vi "Stage v2.vi"() -> ()   [LabVIEW 2025]
uses:
  upper limit.ctl
  lower limit.ctl
  libximc.lvlib
panel:
  in  "Copy Positions":bool
  out "X/256":i32
  out "Z/256":i32
  out "Y/256":i32
  in  "Zero":bool
  in  "Go Home":bool
  in  "Tab Control":T1(tab)=enum."Shift Stage"
  in  "Controller 3":u16(ring) items=["xi-com:\\\\.\\COM4", "xi-com:\\\\.\\COM5", "xi-com:\\\\.\\COM6"]
  in  "Controller 2":u16(ring) items=["xi-com:\\\\.\\COM4", "xi-com:\\\\.\\COM5", "xi-com:\\\\.\\COM6"]
  in  "Controller 1":u16(ring) items=["xi-com:\\\\.\\COM4", "xi-com:\\\\.\\COM5", "xi-com:\\\\.\\COM6"]
  out "s/n 1":u32
  out "s/n 3":u32
  out "s/n 2":u32
  in  "Destination Y":i32
  in  "Destination Z":i32
  in  "Destination X":i32
  in  "Move To Destination":bool
  in  "Update Position":bool
  in  "Move Relative":bool
  in  "Shift Y":i32
  in  "Shift Z":i32
  in  "Shift X":i32
  in  "Shift Amount (Steps)":i32
  in  "shift stage":bool
  in  "Exit":bool
  out "Cursor X":dbl format="%#.2f"
  out "Cursor Z":dbl format="%#.2f"
  out "Cursor Y":dbl format="%#.2f"
  # "Position Status"
  # "Note: units of all positions are in steps."
  # "Initializes each motor in XILab."
  # "Controller IDs"
  # "Serial Numbers"
  # "Moves individual motors to desired height (units in steps)."
  # "Moves individual motors a number of steps."
  # "Moves all three motors the same amount of steps."
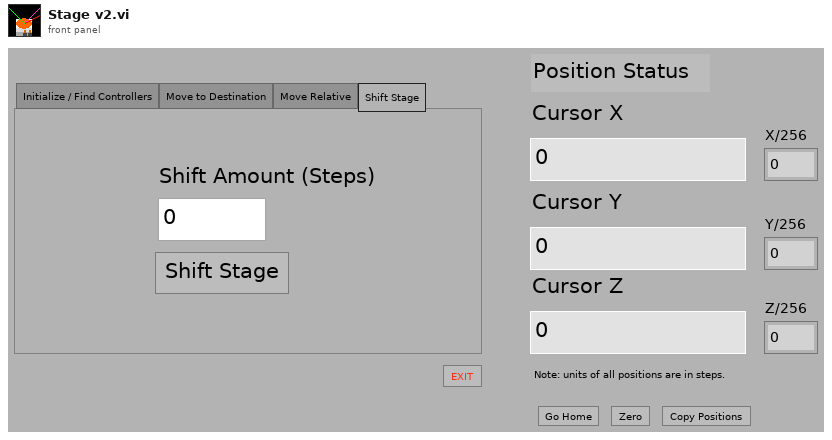
[diagram p1: front panel]
types:
  T1 = enum32{"Initialize / Find Controllers", "Move to Destination", "Move Relative", "Shift Stage"}
  T2 = enum32{"invalid app kind", "Development System", "Run Time System", "Student Edition", "Embedded LabVIEW", "Evaluation", "Custom"}
  T3 = cluster{"Number of controllers":i32, "Controllers' names":string[], "variant":variant, "quit":bool, "IDs":i32[]}
  T4 = typedef "eventvkey.ctl" = enum16{"ASCII", "Enter", "Return", "Shift", "Ctrl", "Alt", "Cmd", "Opt", "Caps", "NumLock", "Clear", "Break", "Up", "Down", "Left", "Right", "Insert", "Delete", "Home", "End", "PageUp", "PageDown", "Escape", "Help", "Pause", "ScrollLock", "F1", "F2", "F3", "F4", "F5", "F6", "F7", "F8", "F9", "F10", "F11", "F12", "F13", "F14", "F15", "F16", "F17", "F18", "F19", "F20", "F21", "F22", "F23", "F24", "Play", "VolumeUp", "VolumeDown", "Mute", "Two Byte Char"}
  T5 = typedef "lower limit.ctl" = i32
  T6 = typedef "upper limit.ctl" = i32
  T7 = cluster{"MoveSts":u32, "MvCmdSts":u32, "PWRSts":u32, "EncSts":u32, "WindSts":u32, "CurPosition":i32, "uCurPosition":i32, "@dummy control@":i8, "@dummy control@":i8, "@dummy control@":i8, "@dummy control@":i8, "EncPosition":i64, "CurSpeed":i32, "uCurSpeed":i32, "Ipwr":i32, "Upwr":i32, "Iusb":i32, "Uusb":i32, "CurT":i32, "Flags":u32, "GPIOFlags":u32, "CmdBufFreeSpace":u32}
  T8 = cluster{"Shift Y":i32, "Shift Z":i32, "Shift X":i32}
  T9 = cluster{"Destination Y":i32, "Destination Z":i32, "Destination X":i32}
  T10 = cluster{"Shift Amount (Steps)":i32, "Shift Amount (Steps)":i32, "Shift Amount (Steps)":i32}
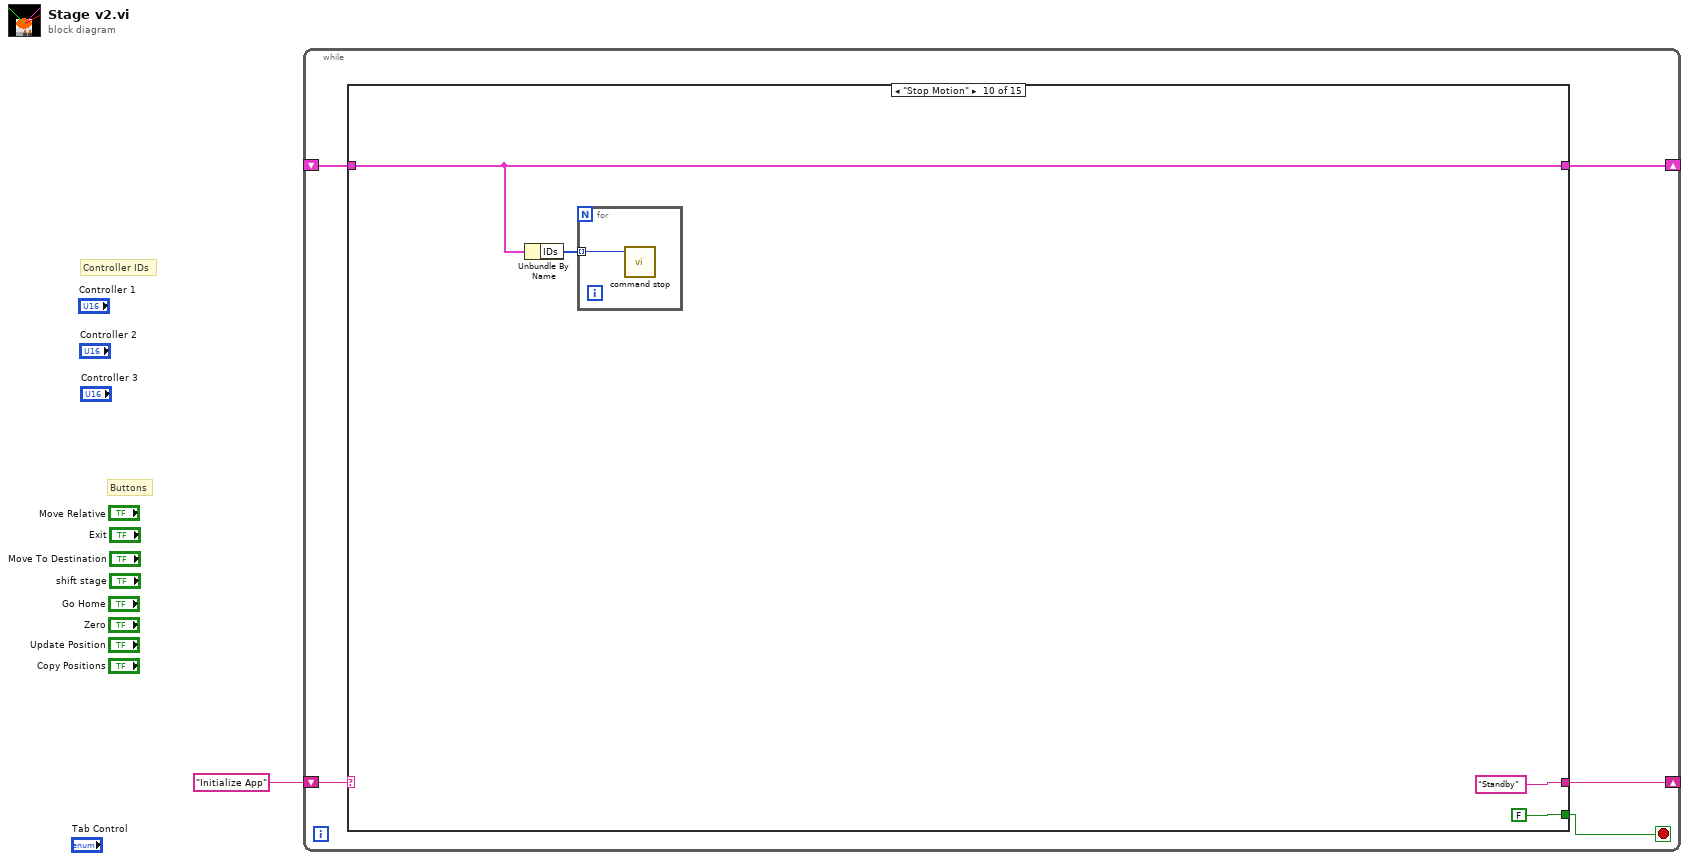
[diagram p0: block diagram]
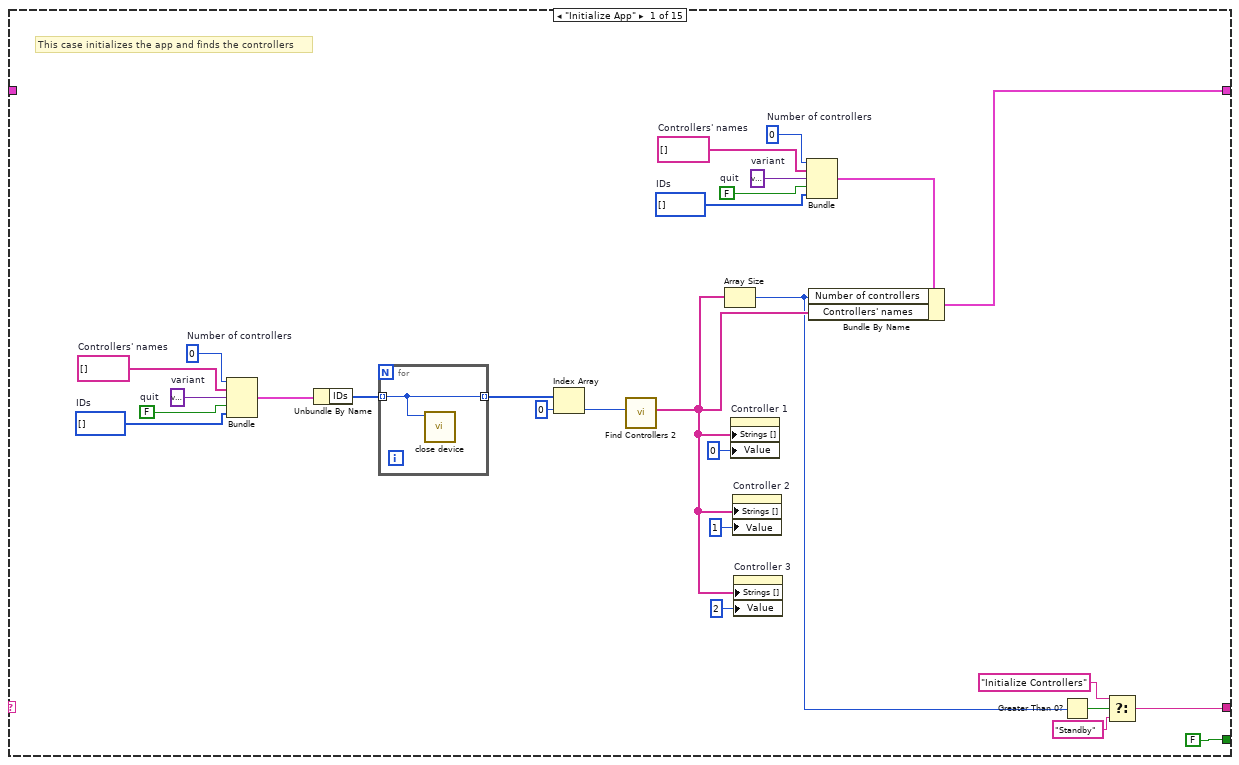
[diagram p2: hidden frame]
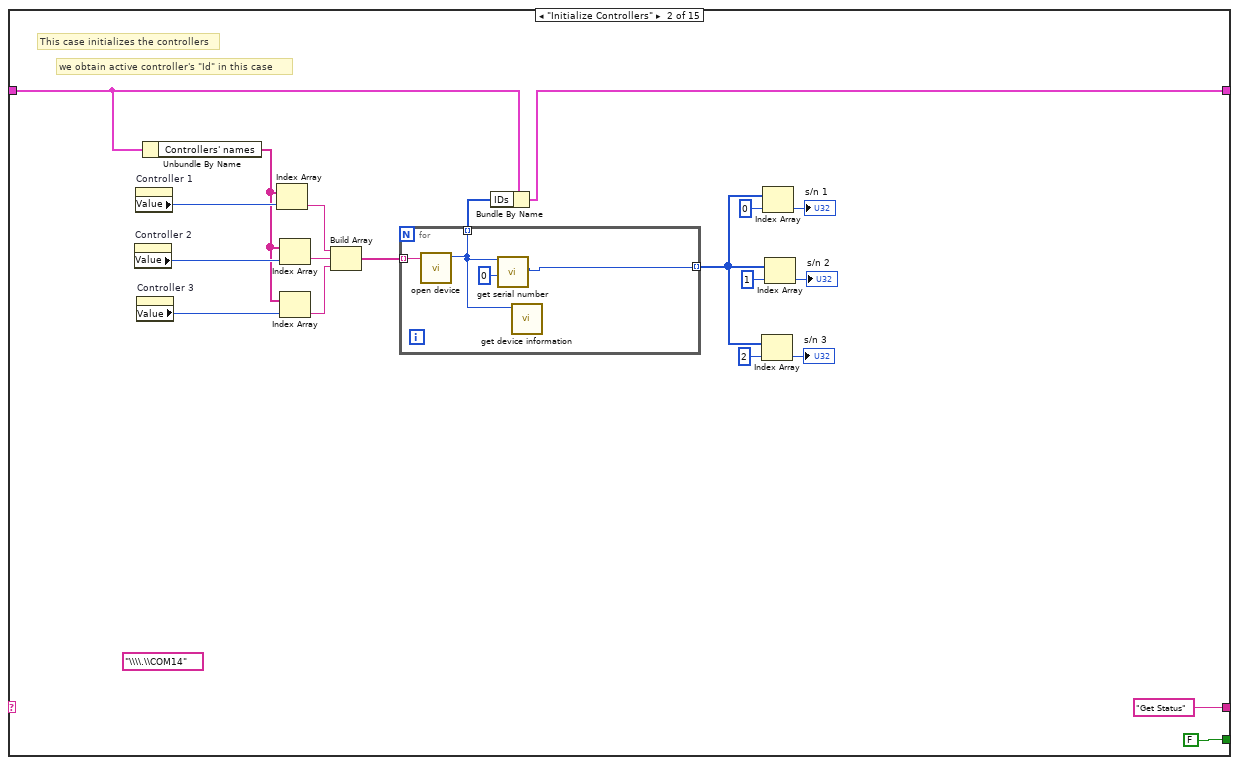
[diagram p3: hidden frame]
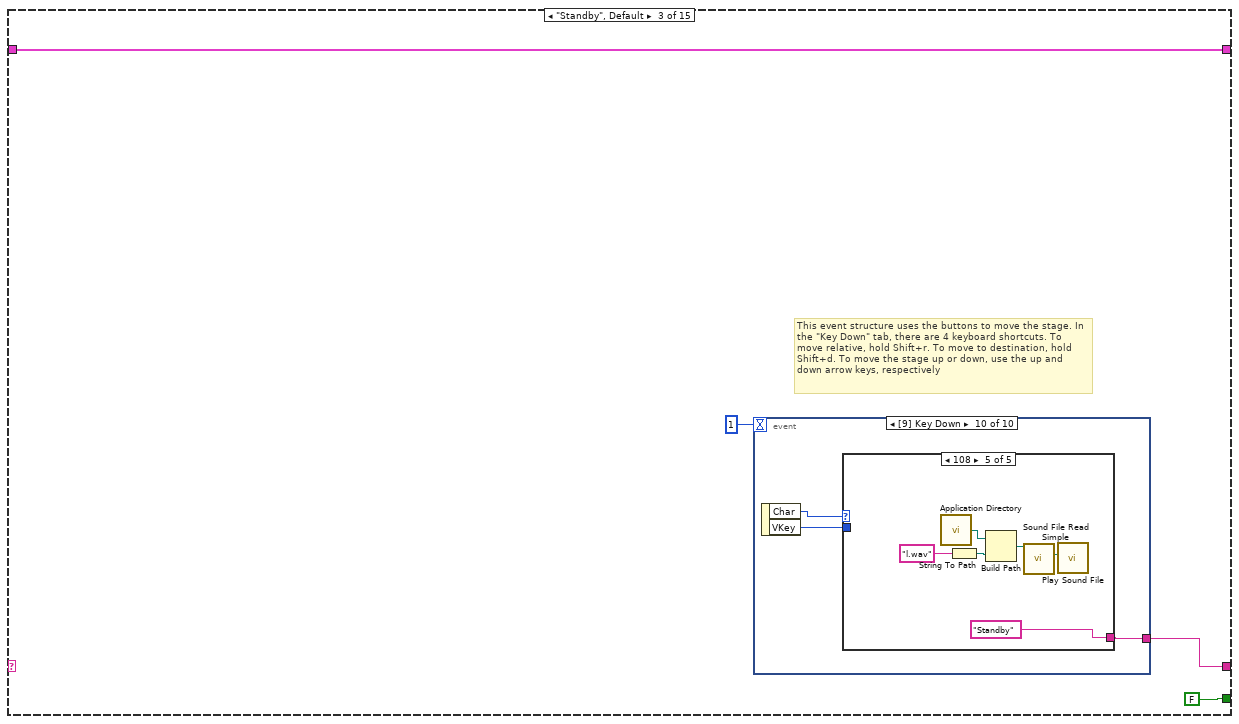
[diagram p4: hidden frame]
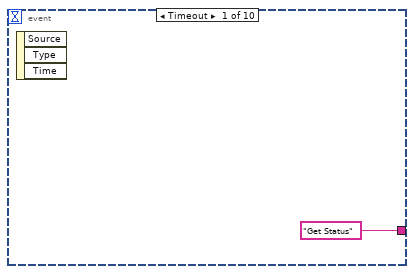
[diagram p5: hidden frame]
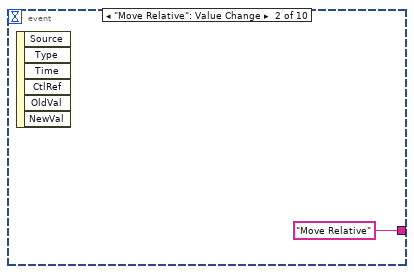
[diagram p6: hidden frame]
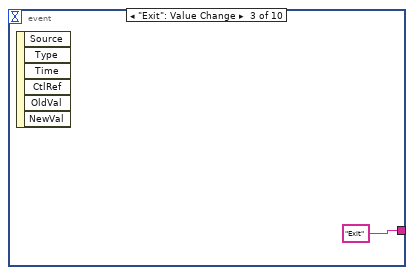
[diagram p7: hidden frame]
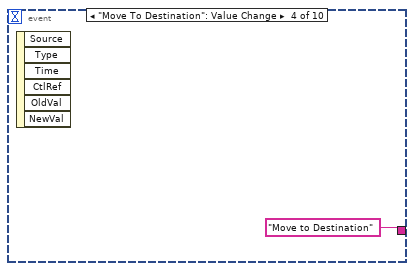
[diagram p8: hidden frame]
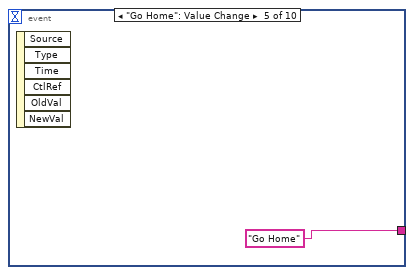
[diagram p9: hidden frame]
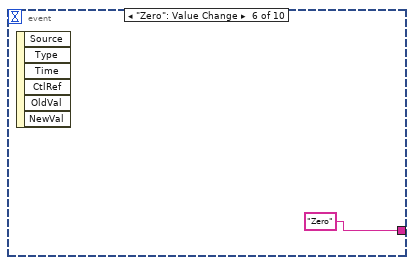
[diagram p10: hidden frame]
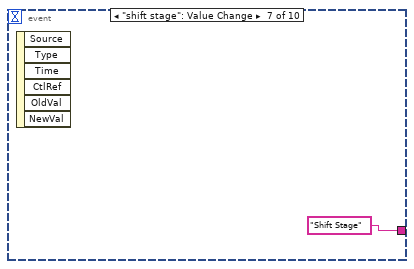
[diagram p11: hidden frame]
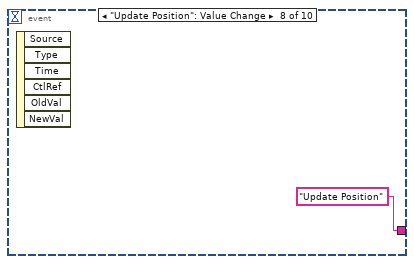
[diagram p12: hidden frame]
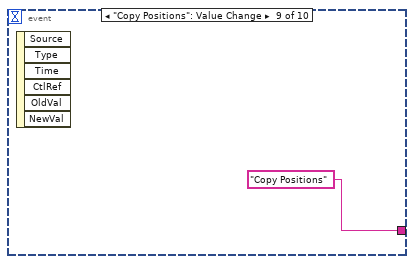
[diagram p13: hidden frame]
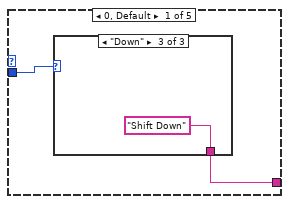
[diagram p14: hidden frame]
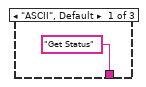
[diagram p15: hidden frame]
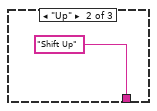
[diagram p16: hidden frame]
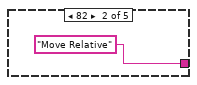
[diagram p17: hidden frame]
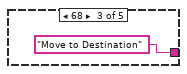
[diagram p18: hidden frame]
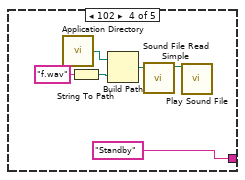
[diagram p19: hidden frame]
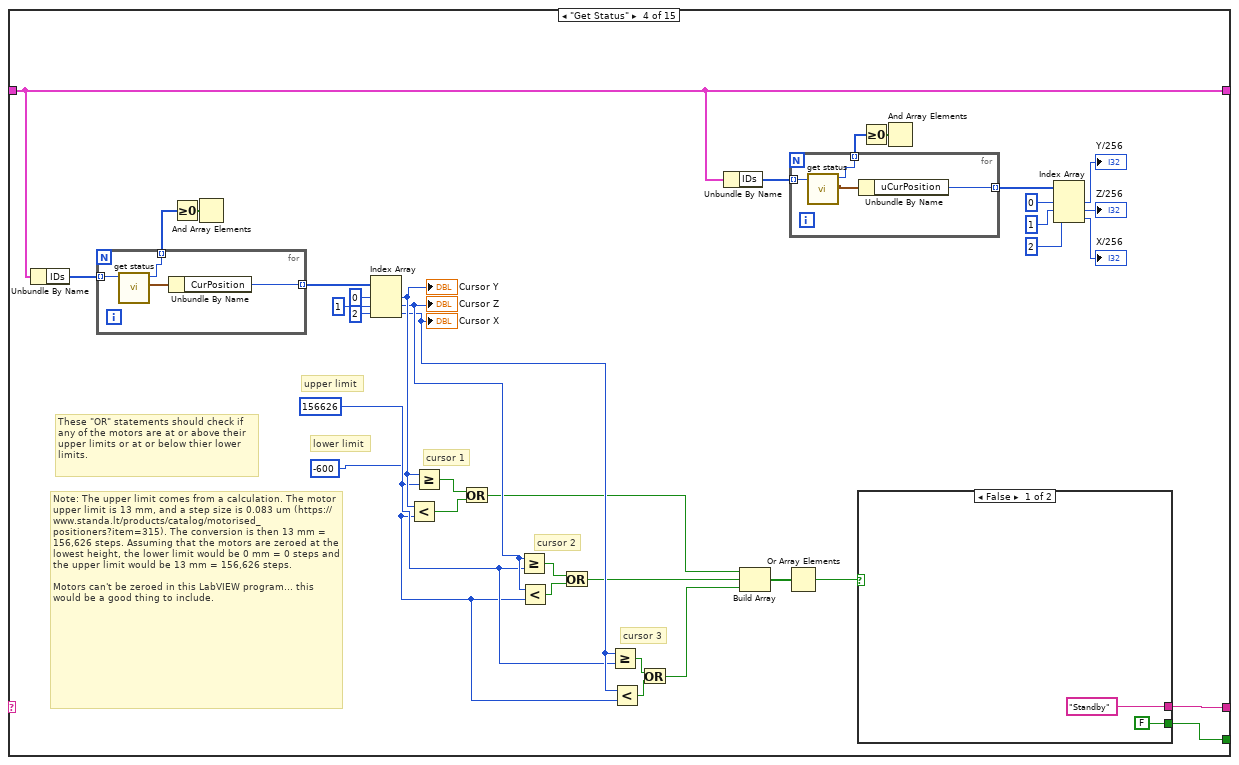
[diagram p20: hidden frame]
diagram:
  # "Buttons"
  # "Controller IDs"
  n1 = while {
    shift-right: [w5] -> _
    shift-left: _ -> [w6]
    shift-right: [w4] -> _
    shift-left: "Initialize App" -> [w3]
    stop <- w2 stop-if-true
    n2 = case shown="\"Stop Motion\"" w3 {
      tunnel: [w27 w44 w62 w94 w151 w213 w262 w320 w380 w430 w435 w440 w448 w470 w478] -> w5
      tunnel: w6 -> [_ w45 w62 w94 w151 w212 w262 w320 w380 w430 w435 w440 w448 w470 w478]
      tunnel: [w8 "Get Status" w60 w119 w150 w211 w261 w319 w379 "Standby" "Standby" "Standby" "Standby" "Standby" "Standby"] -> w4
      tunnel: [FALSE ("quit") FALSE ("quit") FALSE ("quit") w106 FALSE ("quit") FALSE ("quit") FALSE FALSE FALSE FALSE FALSE FALSE FALSE FALSE TRUE ("quit")] -> w2
      frame "Initialize App" {
        w14 = i32[] []  # IDs
        w15 = FALSE  # quit
        w16 = variant  # variant
        w17 = string[] []  # Controllers' names
        w18 = 0  # Number of controllers
        w29 = i32[] []  # IDs
        w30 = FALSE  # quit
        w31 = variant  # variant
        w32 = string[] []  # Controllers' names
        w33 = 0  # Number of controllers
        # "This case initializes the app and finds the controllers"
        n3 = Bundle("Number of controllers"=w18, "Controllers' names"=w17, "variant"=w16, "quit"=w15, "IDs"=w14) -> (w13:T3)  [unwired: 1 in]
        n4 = Unbundle By Name(w13) -> ("IDs"=w20:i32[])
        n5 = for {
          tunnel: w20 -> [w34] mode=indexing
          tunnel: [w34] -> w19 mode=indexing
          n6 = call "close device.vi"("id"=w34) -> ()  [unwired: 8 in, 3 out]
        }
        n7 = Index Array(array=w19, index=0) -> (element=w25:i32)
        n8 = call "Find Controllers 2.vi"("Numeric"=w25) -> ("Names"=w21:string[])  [unwired: 9 in, 1 out]
        n9 = Array Size(array=w21) -> (size(s)=w11:i32)
        n10 = property on="Controller 1" class="Ring (strict)"("Strings []"=w21, "Value"=0) -> ()  [unwired: 2 in, 2 out]
        n11 = property on="Controller 2" class="Ring (strict)"("Strings []"=w21, "Value"=1) -> ()  [unwired: 2 in, 2 out]
        n12 = property on="Controller 3" class="Ring (strict)"("Strings []"=w21, "Value"=2 ("Controller 3")) -> ()  [unwired: 2 in, 2 out]
        n13 = Bundle("Number of controllers"=w33, "Controllers' names"=w32, "variant"=w31, "quit"=w30, "IDs"=w29) -> (w28:T3)  [unwired: 1 in]
        n14 = Bundle By Name(cluster=w28, "Number of controllers"=w11, "Controllers' names"=w21) -> (w27:T3)
        n15 = Greater Than 0?(x=w11) -> (x > 0?=w12:bool)
        n16 = Select(t="Initialize Controllers", s=w12, f="Standby") -> (s? t:f=w8:string)
      }
      frame "Initialize Controllers" {
        (unwired) "\\\\.\\COM14" ("name")
        # "we obtain active controller's \"Id\" in this case"
        # "This case initializes the controllers"
        n17 = property on="Controller 2" class="Ring (strict)"() -> ("Value"=w53:u16)  [unwired: 2 in, 2 out]
        n18 = property on="Controller 1" class="Ring (strict)"() -> ("Value"=w54:u16)  [unwired: 2 in, 2 out]
        n19 = property on="Controller 3" class="Ring (strict)"() -> ("Value"=w52:u16)  [unwired: 2 in, 2 out]
        n20 = Unbundle By Name(w45) -> ("Controllers' names"=w48:string[])
        n21 = Index Array(array=w48, index=w54) -> (element=w49:string)
        n22 = Index Array(array=w48, index=w53) -> (element=w50:string)
        n23 = Index Array(array=w48, index=w52) -> (element=w51:string)
        n24 = Build Array(w49, w50, w51) -> (w47:string[])
        n25 = for {
          tunnel: w47 -> [w58] mode=indexing
          tunnel: [w56] -> w46 mode=indexing
          tunnel: [w55] -> w37 mode=indexing
          n26 = call "open device.vi"("uri"=w58) -> ("function return"=w56:i32)  [unwired: 9 in, 1 out]
          n27 = call "get serial number.vi"("SerialNumber"=0, "id"=w56) -> ("SerialNumber out"=w55:u32)  [unwired: 7 in, 2 out]
          n28 = call "get device information.vi"("id"=w56) -> ()  [unwired: 8 in, 3 out]
        }
        n29 = Bundle By Name(cluster=w45, "IDs"=w46) -> (w44:T3)
        n30 = Index Array(array=w37, index=u32 2 ("serial")) -> (element=→"s/n 3":u32)
        n31 = Index Array(array=w37, index=u32 0 ("serial")) -> (element=→"s/n 1":u32)
        n32 = Index Array(array=w37, index=u32 1 ("serial")) -> (element=→"s/n 2":u32)
      }
      frame "Standby", Default {
        # "This event structure uses the buttons to move the stage. In the \"Key Down\" tab, there are 4 keyboard shortcuts. To move relative, hold Shift+r. To move to destination, hold Shift+d. To move the stage up or down, use the up and down arrow keys, respectively"
        n33 = event shown="[9] Key Down" {
          selector: _ -> [_ _ _ _ _ _ _ _ _ _]
          dyn-events: _ -> [_ _ _ _ _ _ _ _ _ _]
          timeout: 1 -> [_ _ _ _ _ _ _ _ _ _]
          tunnel: ["Get Status" "Move Relative" "Exit" "Move to Destination" "Go Home" "Zero" "Shift Stage" "Update Position" "Copy Positions" w74] -> w60
          event Timeout {
            n34 = event-data() -> ()  [unwired: 1 in, 3 out]
          }
          event "Move Relative": Value Change {
            n35 = event-data() -> ()  [unwired: 1 in, 6 out]
          }
          event "Exit": Value Change {
            n36 = event-data() -> ()  [unwired: 1 in, 6 out]
          }
          event "Move To Destination": Value Change {
            n37 = event-data() -> ()  [unwired: 1 in, 6 out]
          }
          event "Go Home": Value Change {
            n38 = event-data() -> ()  [unwired: 1 in, 6 out]
          }
          event "Zero": Value Change {
            n39 = event-data() -> ()  [unwired: 1 in, 6 out]
          }
          event "shift stage": Value Change {
            n40 = event-data() -> ()  [unwired: 1 in, 6 out]
          }
          event "Update Position": Value Change {
            n41 = event-data() -> ()  [unwired: 1 in, 6 out]
          }
          event "Copy Positions": Value Change {
            n42 = event-data() -> ()  [unwired: 1 in, 6 out]
          }
          event Key Down {
            n43 = event-data() -> ("Char"=w73:i16, "VKey"=w72:T4)  [unwired: 1 in]
            n44 = case shown="108" w73 {
              tunnel: [w75 "Move Relative" "Move to Destination" "Standby" "Standby"] -> w74
              tunnel: w72 -> [w76 _ _ _ _]
              frame 0, Default {
                n45 = case shown="\"Down\"" w76 {
                  tunnel: ["Get Status" "Shift Up" "Shift Down"] -> w75
                  frame "ASCII", Default {
                  }
                  frame "Up" {
                  }
                  frame "Down" {
                  }
                }
              }
              frame 82 {
              }
              frame 68 {
              }
              frame 102 {
                n46 = call <vilib>:"Application Directory.vi"() -> ("Application Directory"=w86:path)
                n47 = String To Path(string="f.wav") -> (path=w84:path)
                n48 = Build Path(base path=w86, name or relative path=w84) -> (appended path=w83:path)
                n49 = call <vilib>:"Sound File Read Simple.vi"("path"=w83) -> ("path out"=w82:path)  [unwired: 7 in, 3 out]
                n50 = call <vilib>:"Play Sound File.vi"("path"=w82) -> ()  [unwired: 9 in, 2 out]
              }
              frame 108 {
                n51 = call <vilib>:"Application Directory.vi"() -> ("Application Directory"=w92:path)
                n52 = String To Path(string="l.wav") -> (path=w90:path)
                n53 = Build Path(base path=w92, name or relative path=w90) -> (appended path=w89:path)
                n54 = call <vilib>:"Sound File Read Simple.vi"("path"=w89) -> ("path out"=w88:path)  [unwired: 7 in, 3 out]
                n55 = call <vilib>:"Play Sound File.vi"("path"=w88) -> ()  [unwired: 9 in, 2 out]
              }
            }
          }
        }
      }
      frame "Get Status" {
        w105 = T5 -600
        w107 = T6 156626
        # "cursor 3"
        # "cursor 2"
        # "cursor 1"
        # "lower limit"
        # "upper limit"
        # "Note: The upper limit comes from a calculation. The motor upper limit is 13 mm, and a step size is 0.083 um (https://www.standa.lt/products/catalog/motorised_positioners?item=315). The conversion is then 13 mm = 156,626 steps. Assuming that the motors are zeroed at the lowest height, the lower limit would be 0 mm = 0 steps and the upper limit would be 13 mm = 156,626 steps.\n\nMotors can't be zeroed in this LabVIEW program... this would be a good thing to include."
        # "These \"OR\" statements should check if any of the motors are at or above their upper limits or at or below thier lower limits."
        n56 = Unbundle By Name(w94) -> ("IDs"=w129:i32[])
        n57 = for {
          tunnel: [w147] -> w127 mode=indexing
          tunnel: w129 -> [w146] mode=indexing
          tunnel: [w145] -> w128 mode=indexing
          n58 = call "get status.vi"("id"=w146) -> ("status out"=w144:T7, "function return"=w145:i32)  [unwired: 8 in, 1 out]
          n59 = Unbundle By Name(w144) -> ("CurPosition"=w147:i32)
        }
        n60 = Greater Or Equal To 0?(x=w128) -> (x >= 0?=w123:bool[])
        n61 = And Array Elements(Boolean array=w123) -> ()  [unwired: 1 out]
        n62 = Index Array(array=w127, index #1=0 ("index"), index #2=1 ("index"), index #3=2 ("index")) -> (element #1=w121:i32, element #2=w114:i32, element #3=w113:i32)
        "Cursor Y" <- w121
        "Cursor Z" <- w114
        "Cursor X" <- w113
        n63 = Less?(x=w121, y=w105) -> (x < y?=w120:bool)
        n64 = Greater Or Equal?(x=w121, y=w107) -> (x >= y?=w122:bool)
        n65 = Or(x=w122, y=w120) -> (x .or. y?=w112:bool)
        n66 = Greater Or Equal?(x=w114, y=w107) -> (x >= y?=w118:bool)
        n67 = Less?(x=w114, y=w105) -> (x < y?=w117:bool)
        n68 = Or(x=w118, y=w117) -> (x .or. y?=w111:bool)
        n69 = Greater Or Equal?(x=w113, y=w107) -> (x >= y?=w116:bool)
        n70 = Less?(x=w113, y=w105) -> (x < y?=w115:bool)
        n71 = Or(x=w116, y=w115) -> (x .or. y?=w110:bool)
        n72 = Unbundle By Name(w94) -> ("IDs"=w104:i32[])
        n73 = Build Array(w112, w111, w110) -> (w109:bool[])
        n74 = Or Array Elements(Boolean array=w109) -> (logical OR=w108:bool)
        n75 = for {
          tunnel: [w133] -> w102 mode=indexing
          tunnel: w104 -> [w132] mode=indexing
          tunnel: [w131] -> w103 mode=indexing
          n76 = call "get status.vi"("id"=w132) -> ("status out"=w130:T7, "function return"=w131:i32)  [unwired: 8 in, 1 out]
          n77 = Unbundle By Name(w130) -> ("uCurPosition"=w133:i32)
        }
        n78 = case shown="False" w108 {
          tunnel: ["Standby" "Stop Motion"] -> w119
          tunnel: [FALSE w141] -> w106
          frame False {
          }
          frame True {
            # "If any of them move past the limits, the program will stop. You won't be able to use this LabVIEW program until the height is fixed in XILab."
            n79 = call <vilib>:"Application Directory.vi"() -> ("Application Directory"=w140:path)
            n80 = String To Path(string="l.wav") -> (path=w138:path)
            n81 = Build Path(base path=w140, name or relative path=w138) -> (appended path=w137:path)
            n82 = call <vilib>:"Sound File Read Simple.vi"("path"=w137) -> ("path out"=w136:path)  [unwired: 7 in, 3 out]
            n83 = call <vilib>:"Play Sound File.vi"("path"=w136) -> ()  [unwired: 9 in, 2 out]
            n84 = One Button Dialog(message="You've gone too far this time...\nPlease check the height of the stage and move it back to a normal height using XILab <3") -> (true=w141:bool)  [unwired: 1 in]
          }
        }
        n85 = Greater Or Equal To 0?(x=w103) -> (x >= 0?=w101:bool[])
        n86 = And Array Elements(Boolean array=w101) -> ()  [unwired: 1 out]
        n87 = Index Array(array=w102, index #1=0 ("index"), index #2=1 ("index"), index #3=2 ("index")) -> (element #1=→"Y/256":i32, element #2=→"Z/256":i32, element #3=→"X/256":i32)
      }
      frame "Move Relative" {
        w148 = T6 156626
        w149 = -1
        # "cursor 3"
        # "cursor 2"
        # "cursor 1"
        # "lower limit"
        # "upper limit"
        n88 = Unbundle By Name(w151) -> ("IDs"=w178:i32[])
        n89 = for {
          tunnel: [w205] -> w176 mode=indexing
          tunnel: w178 -> [w204] mode=indexing
          tunnel: [w203] -> w177 mode=indexing
          n90 = call "get status.vi"("id"=w204) -> ("status out"=w202:T7, "function return"=w203:i32)  [unwired: 8 in, 1 out]
          n91 = Unbundle By Name(w202) -> ("CurPosition"=w205:i32)
        }
        n92 = Greater Or Equal To 0?(x=w177) -> (x >= 0?=w172:bool[])
        n93 = And Array Elements(Boolean array=w172) -> ()  [unwired: 1 out]
        n94 = Index Array(array=w176, index #1=0 ("index"), index #2=1 ("index"), index #3=2 ("index")) -> (element #1=w160:i32, element #2=w159:i32, element #3=w158:i32)
        n95 = Add(x="Shift Y", y=w160) -> (x+y=w157:i32)
        n96 = Add(x="Shift Z", y=w159) -> (x+y=w155:i32)
        n97 = Add(x="Shift X", y=w158) -> (x+y=w156:i32)
        n98 = Less Or Equal?(x=w157, y=w149) -> (x <= y?=w170:bool)
        n99 = Greater Or Equal?(x=w156, y=w148) -> (x >= y?=w167:bool)
        n100 = Greater Or Equal?(x=w157, y=w148) -> (x >= y?=w171:bool)
        n101 = Greater Or Equal?(x=w155, y=w148) -> (x >= y?=w169:bool)
        n102 = Less Or Equal?(x=w155, y=w149) -> (x <= y?=w168:bool)
        n103 = Less Or Equal?(x=w156, y=w149) -> (x <= y?=w166:bool)
        n104 = Or(x=w167, y=w166) -> (x .or. y?=w163:bool)
        n105 = Or(x=w169, y=w168) -> (x .or. y?=w164:bool)
        n106 = Or(x=w171, y=w170) -> (x .or. y?=w165:bool)
        n107 = Build Array(w165, w164, w163) -> (w162:bool[])
        n108 = Or Array Elements(Boolean array=w162) -> (logical OR=w161:bool)
        n109 = case shown="False" w161 {
          tunnel: ["Standby" "Stop Motion"] -> w150
          tunnel: "Shift Y" -> [w190 _]
          tunnel: "Shift Z" -> [w189 _]
          tunnel: "Shift X" -> [w188 _]
          tunnel: w151 -> [w187 w199]
          tunnel: [w185 w199] -> _
          frame False {
            n110 = Bundle("Shift Y"=w190, "Shift Z"=w189, "Shift X"=w188) -> (w186:T8)  [unwired: 1 in]
            n111 = Bundle By Name(cluster=w187, "variant"=w186) -> (w185:T3)
            n112 = Unbundle By Name(w185) -> ("IDs"=w180:i32[], "variant"=w182:variant)
            n113 = Variant To Data(type=cluster{u32, u32, u32} {0, 0, 0}, Variant=w182) -> (data=w183:cluster{u32, u32, u32})  [unwired: 1 in, 1 out]
            n114 = Cluster To Array(cluster=w183) -> (array=w184:u32[])
            n115 = for {
              tunnel: w184 -> [w192] mode=indexing
              tunnel: w180 -> [w193] mode=indexing
              n116 = call "command movr.vi"("DeltaPosition"=w192, "id"=w193) -> ()  [unwired: 8 in, 2 out]
            }
          }
          frame True {
            # "If any of them move past the limits, the motors won't move."
            n117 = call <vilib>:"Application Directory.vi"() -> ("Application Directory"=w198:path)
            n118 = String To Path(string="l.wav") -> (path=w196:path)
            n119 = Build Path(base path=w198, name or relative path=w196) -> (appended path=w195:path)
            n120 = call <vilib>:"Sound File Read Simple.vi"("path"=w195) -> ("path out"=w194:path)  [unwired: 7 in, 3 out]
            n121 = One Button Dialog(message="You've gone too far this time...\nPlease ensure the step size does not go past the limits <3") -> ()  [unwired: 1 in, 1 out]
            n122 = call <vilib>:"Play Sound File.vi"("path"=w194) -> ()  [unwired: 9 in, 2 out]
          }
        }
      }
      frame "Move to Destination" {
        w206 = T6 156626
        w207 = -1
        # "cursor 3"
        # "cursor 2"
        # "cursor 1"
        # "lower limit"
        # "upper limit"
        n123 = Unbundle By Name(w212) -> ("IDs"=w231:i32[])
        n124 = for {
          tunnel: [w258] -> w229 mode=indexing
          tunnel: w231 -> [w257] mode=indexing
          tunnel: [w256] -> w230 mode=indexing
          n125 = call "get status.vi"("id"=w257) -> ("status out"=w255:T7, "function return"=w256:i32)  [unwired: 8 in, 1 out]
          n126 = Unbundle By Name(w255) -> ("CurPosition"=w258:i32)
        }
        n127 = Greater Or Equal To 0?(x=w230) -> (x >= 0?=w225:bool[])
        n128 = And Array Elements(Boolean array=w225) -> ()  [unwired: 1 out]
        n129 = Index Array(array=w229, index #1=0 ("index"), index #2=1 ("index"), index #3=2 ("index")) -> ()  [unwired: 3 out]
        n130 = Less Or Equal?(x="Destination Y", y=w207) -> (x <= y?=w223:bool)
        n131 = Greater Or Equal?(x="Destination X", y=w206) -> (x >= y?=w220:bool)
        n132 = Greater Or Equal?(x="Destination Y", y=w206) -> (x >= y?=w224:bool)
        n133 = Greater Or Equal?(x="Destination Z", y=w206) -> (x >= y?=w222:bool)
        n134 = Less Or Equal?(x="Destination Z", y=w207) -> (x <= y?=w221:bool)
        n135 = Less Or Equal?(x="Destination X", y=w207) -> (x <= y?=w219:bool)
        n136 = Or(x=w220, y=w219) -> (x .or. y?=w216:bool)
        n137 = Or(x=w222, y=w221) -> (x .or. y?=w217:bool)
        n138 = Or(x=w224, y=w223) -> (x .or. y?=w218:bool)
        n139 = Build Array(w218, w217, w216) -> (w215:bool[])
        n140 = Or Array Elements(Boolean array=w215) -> (logical OR=w214:bool)
        n141 = case shown="False" w214 {
          tunnel: ["Standby" "Stop Motion"] -> w211
          tunnel: "Destination Y" -> [w237 _]
          tunnel: "Destination Z" -> [w236 _]
          tunnel: "Destination X" -> [w235 _]
          tunnel: w212 -> [w234 w252]
          tunnel: [w233 w252] -> w213
          frame False {
            n142 = Bundle("Destination Y"=w237, "Destination Z"=w236, "Destination X"=w235) -> (w239:T9)  [unwired: 1 in]
            n143 = Bundle By Name(cluster=w234, "variant"=w239) -> (w233:T3)
            n144 = Unbundle By Name(w233) -> ("IDs"=w241:i32[], "variant"=w243:variant)
            n145 = Variant To Data(type=cluster{u32, u32, u32} {0, 0, 0}, Variant=w243) -> (data=w240:cluster{u32, u32, u32})  [unwired: 1 in, 1 out]
            n146 = Cluster To Array(cluster=w240) -> (array=w242:u32[])
            n147 = for {
              tunnel: w242 -> [w245] mode=indexing
              tunnel: w241 -> [w246] mode=indexing
              n148 = call "command move.vi"("Position"=w245, "id"=w246) -> ()  [unwired: 8 in, 2 out]
            }
          }
          frame True {
            # "If any of them move past the limits, the motors won't move."
            n149 = call <vilib>:"Application Directory.vi"() -> ("Application Directory"=w251:path)
            n150 = String To Path(string="l.wav") -> (path=w249:path)
            n151 = Build Path(base path=w251, name or relative path=w249) -> (appended path=w248:path)
            n152 = call <vilib>:"Sound File Read Simple.vi"("path"=w248) -> ("path out"=w247:path)  [unwired: 7 in, 3 out]
            n153 = call <vilib>:"Play Sound File.vi"("path"=w247) -> ()  [unwired: 9 in, 2 out]
            n154 = One Button Dialog(message="You've gone too far this time...\nPlease ensure the step size does not go past the limits <3") -> ()  [unwired: 1 in, 1 out]
          }
        }
      }
      frame "Shift Stage" {
        w259 = T6 156626
        w260 = -1
        # "cursor 3"
        # "cursor 2"
        # "cursor 1"
        # "lower limit"
        # "upper limit"
        n155 = Unbundle By Name(w262) -> ("IDs"=w287:i32[])
        n156 = for {
          tunnel: [w314] -> w285 mode=indexing
          tunnel: w287 -> [w313] mode=indexing
          tunnel: [w312] -> w286 mode=indexing
          n157 = call "get status.vi"("id"=w313) -> ("status out"=w311:T7, "function return"=w312:i32)  [unwired: 8 in, 1 out]
          n158 = Unbundle By Name(w311) -> ("CurPosition"=w314:i32)
        }
        n159 = Greater Or Equal To 0?(x=w286) -> (x >= 0?=w281:bool[])
        n160 = And Array Elements(Boolean array=w281) -> ()  [unwired: 1 out]
        n161 = Index Array(array=w285, index #1=0 ("index"), index #2=1 ("index"), index #3=2 ("index")) -> (element #1=w269:i32, element #2=w268:i32, element #3=w267:i32)
        n162 = Add(x="Shift Amount (Steps)", y=w269) -> (x+y=w266:i32)
        n163 = Add(x="Shift Amount (Steps)", y=w268) -> (x+y=w264:i32)
        n164 = Add(x="Shift Amount (Steps)", y=w267) -> (x+y=w265:i32)
        n165 = Less Or Equal?(x=w266, y=w260) -> (x <= y?=w279:bool)
        n166 = Greater Or Equal?(x=w265, y=w259) -> (x >= y?=w276:bool)
        n167 = Greater Or Equal?(x=w266, y=w259) -> (x >= y?=w280:bool)
        n168 = Greater Or Equal?(x=w264, y=w259) -> (x >= y?=w278:bool)
        n169 = Less Or Equal?(x=w264, y=w260) -> (x <= y?=w277:bool)
        n170 = Less Or Equal?(x=w265, y=w260) -> (x <= y?=w275:bool)
        n171 = Or(x=w276, y=w275) -> (x .or. y?=w272:bool)
        n172 = Or(x=w278, y=w277) -> (x .or. y?=w273:bool)
        n173 = Or(x=w280, y=w279) -> (x .or. y?=w274:bool)
        n174 = Build Array(w274, w273, w272) -> (w271:bool[])
        n175 = Or Array Elements(Boolean array=w271) -> (logical OR=w270:bool)
        n176 = case shown="False" w270 {
          tunnel: ["Standby" "Stop Motion"] -> w261
          tunnel: "Shift Amount (Steps)" -> [w299 _]
          tunnel: "Shift Amount (Steps)" -> [w298 _]
          tunnel: "Shift Amount (Steps)" -> [w297 _]
          tunnel: w262 -> [w296 w308]
          tunnel: [w294 w308] -> _
          frame False {
            n177 = Bundle("Shift Amount (Steps)"=w299, "Shift Amount (Steps)"=w298, "Shift Amount (Steps)"=w297) -> (w295:T10)  [unwired: 1 in]
            n178 = Bundle By Name(cluster=w296, "variant"=w295) -> (w294:T3)
            n179 = Unbundle By Name(w294) -> ("IDs"=w289:i32[], "variant"=w291:variant)
            n180 = Variant To Data(type=cluster{u32, u32, u32} {0, 0, 0}, Variant=w291) -> (data=w292:cluster{u32, u32, u32})  [unwired: 1 in, 1 out]
            n181 = Cluster To Array(cluster=w292) -> (array=w293:u32[])
            n182 = for {
              tunnel: w293 -> [w301] mode=indexing
              tunnel: w289 -> [w302] mode=indexing
              n183 = call "command movr.vi"("DeltaPosition"=w301, "id"=w302) -> ()  [unwired: 8 in, 2 out]
            }
          }
          frame True {
            # "If any of them move past the limits, the motors won't move."
            n184 = call <vilib>:"Application Directory.vi"() -> ("Application Directory"=w307:path)
            n185 = String To Path(string="l.wav") -> (path=w305:path)
            n186 = Build Path(base path=w307, name or relative path=w305) -> (appended path=w304:path)
            n187 = call <vilib>:"Sound File Read Simple.vi"("path"=w304) -> ("path out"=w303:path)  [unwired: 7 in, 3 out]
            n188 = call <vilib>:"Play Sound File.vi"("path"=w303) -> ()  [unwired: 9 in, 2 out]
            n189 = One Button Dialog(message="You've gone too far this time...\nPlease ensure the step size does not go past the limits <3") -> ()  [unwired: 1 in, 1 out]
          }
        }
      }
      frame "Shift Up" {
        w315 = T6 156626
        w316 = -1
        # "cursor 3"
        # "cursor 2"
        # "cursor 1"
        # "lower limit"
        # "upper limit"
        n190 = Unbundle By Name(w320) -> ("IDs"=w344:i32[])
        n191 = for {
          tunnel: [w371] -> w342 mode=indexing
          tunnel: w344 -> [w370] mode=indexing
          tunnel: [w369] -> w343 mode=indexing
          n192 = call "get status.vi"("id"=w370) -> ("status out"=w368:T7, "function return"=w369:i32)  [unwired: 8 in, 1 out]
          n193 = Unbundle By Name(w368) -> ("CurPosition"=w371:i32)
        }
        n194 = Greater Or Equal To 0?(x=w343) -> (x >= 0?=w338:bool[])
        n195 = And Array Elements(Boolean array=w338) -> ()  [unwired: 1 out]
        n196 = local read "Shift Amount (Steps)"() -> (w317:i32)
        n197 = Index Array(array=w342, index #1=0 ("index"), index #2=1 ("index"), index #3=2 ("index")) -> (element #1=w326:i32, element #2=w325:i32, element #3=w324:i32)
        n198 = Absolute Value(x=w317) -> (abs(x)=w318:i32)
        n199 = Add(x=w318, y=w326) -> (x+y=w323:i32)
        n200 = Add(x=w318, y=w325) -> (x+y=w321:i32)
        n201 = Add(x=w318, y=w324) -> (x+y=w322:i32)
        n202 = Less Or Equal?(x=w323, y=w316) -> (x <= y?=w336:bool)
        n203 = Greater Or Equal?(x=w322, y=w315) -> (x >= y?=w333:bool)
        n204 = Greater Or Equal?(x=w323, y=w315) -> (x >= y?=w337:bool)
        n205 = Greater Or Equal?(x=w321, y=w315) -> (x >= y?=w335:bool)
        n206 = Less Or Equal?(x=w321, y=w316) -> (x <= y?=w334:bool)
        n207 = Less Or Equal?(x=w322, y=w316) -> (x <= y?=w332:bool)
        n208 = Or(x=w333, y=w332) -> (x .or. y?=w329:bool)
        n209 = Or(x=w335, y=w334) -> (x .or. y?=w330:bool)
        n210 = Or(x=w337, y=w336) -> (x .or. y?=w331:bool)
        n211 = Build Array(w331, w330, w329) -> (w328:bool[])
        n212 = Or Array Elements(Boolean array=w328) -> (logical OR=w327:bool)
        n213 = case shown="False" w327 {
          tunnel: ["Standby" "Stop Motion"] -> w319
          tunnel: w318 -> [w356 _]
          tunnel: w318 -> [w355 _]
          tunnel: w318 -> [w354 _]
          tunnel: w320 -> [w353 w365]
          tunnel: [w351 w365] -> _
          frame False {
            n214 = Bundle(w356, w355, w354) -> (w352:cluster{i32, i32, i32})  [unwired: 1 in]
            n215 = Bundle By Name(cluster=w353, "variant"=w352) -> (w351:T3)
            n216 = Unbundle By Name(w351) -> ("IDs"=w346:i32[], "variant"=w348:variant)
            n217 = Variant To Data(type=cluster{u32, u32, u32} {0, 0, 0}, Variant=w348) -> (data=w349:cluster{u32, u32, u32})  [unwired: 1 in, 1 out]
            n218 = Cluster To Array(cluster=w349) -> (array=w350:u32[])
            n219 = for {
              tunnel: w350 -> [w358] mode=indexing
              tunnel: w346 -> [w359] mode=indexing
              n220 = call "command movr.vi"("DeltaPosition"=w358, "id"=w359) -> ()  [unwired: 8 in, 2 out]
            }
          }
          frame True {
            # "If any of them move past the limits, the motors won't move."
            n221 = call <vilib>:"Application Directory.vi"() -> ("Application Directory"=w364:path)
            n222 = String To Path(string="l.wav") -> (path=w362:path)
            n223 = Build Path(base path=w364, name or relative path=w362) -> (appended path=w361:path)
            n224 = call <vilib>:"Sound File Read Simple.vi"("path"=w361) -> ("path out"=w360:path)  [unwired: 7 in, 3 out]
            n225 = call <vilib>:"Play Sound File.vi"("path"=w360) -> ()  [unwired: 9 in, 2 out]
            n226 = One Button Dialog(message="You've gone too far this time...\nPlease ensure the step size does not go past the limits <3") -> ()  [unwired: 1 in, 1 out]
          }
        }
      }
      frame "Shift Down" {
        w372 = T6 156626
        w382 = -1
        # "cursor 3"
        # "cursor 2"
        # "cursor 1"
        # "lower limit"
        # "upper limit"
        n227 = Unbundle By Name(w380) -> ("IDs"=w402:i32[])
        n228 = for {
          tunnel: [w429] -> w400 mode=indexing
          tunnel: w402 -> [w428] mode=indexing
          tunnel: [w427] -> w401 mode=indexing
          n229 = call "get status.vi"("id"=w428) -> ("status out"=w426:T7, "function return"=w427:i32)  [unwired: 8 in, 1 out]
          n230 = Unbundle By Name(w426) -> ("CurPosition"=w429:i32)
        }
        n231 = Greater Or Equal To 0?(x=w401) -> (x >= 0?=w396:bool[])
        n232 = And Array Elements(Boolean array=w396) -> ()  [unwired: 1 out]
        n233 = local read "Shift Amount (Steps)"() -> (w378:i32)
        n234 = Index Array(array=w400, index #1=0 ("index"), index #2=1 ("index"), index #3=2 ("index")) -> (element #1=w377:i32, element #2=w376:i32, element #3=w375:i32)
        n235 = Absolute Value(x=w378) -> (abs(x)=w374:i32)
        n236 = Subtract(x=w377, y=w374) -> (x-y=w384:i32)
        n237 = Subtract(x=w376, y=w374) -> (x-y=w381:i32)
        n238 = Subtract(x=w375, y=w374) -> (x-y=w383:i32)
        n239 = Less Or Equal?(x=w384, y=w382) -> (x <= y?=w394:bool)
        n240 = Greater Or Equal?(x=w383, y=w372) -> (x >= y?=w391:bool)
        n241 = Greater Or Equal?(x=w384, y=w372) -> (x >= y?=w395:bool)
        n242 = Greater Or Equal?(x=w381, y=w372) -> (x >= y?=w393:bool)
        n243 = Less Or Equal?(x=w381, y=w382) -> (x <= y?=w392:bool)
        n244 = Less Or Equal?(x=w383, y=w382) -> (x <= y?=w390:bool)
        n245 = Or(x=w391, y=w390) -> (x .or. y?=w387:bool)
        n246 = Or(x=w393, y=w392) -> (x .or. y?=w388:bool)
        n247 = Or(x=w395, y=w394) -> (x .or. y?=w389:bool)
        n248 = Negate(x=w374) -> (-x=w373:i32)
        n249 = Build Array(w389, w388, w387) -> (w386:bool[])
        n250 = Or Array Elements(Boolean array=w386) -> (logical OR=w385:bool)
        n251 = case shown="False" w385 {
          tunnel: ["Standby" "Stop Motion"] -> w379
          tunnel: w373 -> [w414 _]
          tunnel: w373 -> [w413 _]
          tunnel: w373 -> [w412 _]
          tunnel: w380 -> [w411 w423]
          tunnel: [w409 w423] -> _
          frame False {
            n252 = Bundle(w414, w413, w412) -> (w410:cluster{i32, i32, i32})  [unwired: 1 in]
            n253 = Bundle By Name(cluster=w411, "variant"=w410) -> (w409:T3)
            n254 = Unbundle By Name(w409) -> ("IDs"=w404:i32[], "variant"=w406:variant)
            n255 = Variant To Data(type=cluster{u32, u32, u32} {0, 0, 0}, Variant=w406) -> (data=w407:cluster{u32, u32, u32})  [unwired: 1 in, 1 out]
            n256 = Cluster To Array(cluster=w407) -> (array=w408:u32[])
            n257 = for {
              tunnel: w408 -> [w416] mode=indexing
              tunnel: w404 -> [w417] mode=indexing
              n258 = call "command movr.vi"("DeltaPosition"=w416, "id"=w417) -> ()  [unwired: 8 in, 2 out]
            }
          }
          frame True {
            # "If any of them move past the limits, the motors won't move."
            n259 = call <vilib>:"Application Directory.vi"() -> ("Application Directory"=w422:path)
            n260 = String To Path(string="l.wav") -> (path=w420:path)
            n261 = Build Path(base path=w422, name or relative path=w420) -> (appended path=w419:path)
            n262 = call <vilib>:"Sound File Read Simple.vi"("path"=w419) -> ("path out"=w418:path)  [unwired: 7 in, 3 out]
            n263 = call <vilib>:"Play Sound File.vi"("path"=w418) -> ()  [unwired: 9 in, 2 out]
            n264 = One Button Dialog(message="You've gone too far this time...\nPlease ensure the step size does not go past the limits <3") -> ()  [unwired: 1 in, 1 out]
          }
        }
      }
      frame "Stop Motion" {
        n265 = Unbundle By Name(w430) -> ("IDs"=w431:i32[])
        n266 = for {
          tunnel: w431 -> [w434] mode=indexing
          n267 = call "command stop.vi"("id"=w434) -> ()  [unwired: 9 in, 2 out]
        }
      }
      frame "Go Home" {
        n268 = Unbundle By Name(w435) -> ("IDs"=w436:i32[])
        n269 = for {
          tunnel: w436 -> [w439] mode=indexing
          n270 = call "command home.vi"("id"=w439) -> ()  [unwired: 9 in, 2 out]
        }
      }
      frame "Zero" {
        n271 = Unbundle By Name(w440) -> ("IDs"=w441:i32[])
        n272 = for {
          tunnel: w441 -> [w444] mode=indexing
          n273 = call "command zero.vi"("id"=w444) -> ()  [unwired: 9 in, 2 out]
        }
      }
      frame "Update Position" {
        # "When the \"Update Position\" button is pressed, the cursor destinations in the \"Move to Destination\" tab will populate with the current cursor positions."
        n274 = Unbundle By Name(w448) -> ("IDs"=w455:i32[])
        n275 = for {
          tunnel: [w461] -> w453 mode=indexing
          tunnel: w455 -> [w460] mode=indexing
          tunnel: [w459] -> w454 mode=indexing
          n276 = call "get status.vi"("id"=w460) -> ("status out"=w458:T7, "function return"=w459:i32)  [unwired: 8 in, 1 out]
          n277 = Unbundle By Name(w458) -> ("CurPosition"=w461:i32)
        }
        n278 = Greater Or Equal To 0?(x=w454) -> (x >= 0?=w452:bool[])
        n279 = And Array Elements(Boolean array=w452) -> ()  [unwired: 1 out]
        n280 = Index Array(array=w453, index #1=0 ("index"), index #2=1 ("index"), index #3=2 ("index")) -> (element #1=w445:i32, element #2=w447:i32, element #3=w446:i32)
        n281 = local write "Destination Y"(w445) -> ()
        n282 = local write "Destination Z"(w447) -> ()
        n283 = local write "Destination X"(w446) -> ()
      }
      frame "Copy Positions" {
        # "When \"Copy Positions\" button is pressed, the current cursor values will be copied to the Clipboad. These values can then be pasted in an Excel file."
        n284 = property on="Cursor X" class="DigNum (strict)"() -> ("Value"=w469:dbl)  [unwired: 2 in, 2 out]
        n285 = property on="Cursor Y" class="DigNum (strict)"() -> ("Value"=w468:dbl)  [unwired: 2 in, 2 out]
        n286 = property on="Cursor Z" class="DigNum (strict)"() -> ("Value"=w467:dbl)  [unwired: 2 in, 2 out]
        n287 = Build Array(w469, w468, w467) -> (w466:dbl[])
        n288 = Array To Spreadsheet String(array=w466, 3:"%s" ("initial string")) -> (spreadsheet string=w465:string)  [unwired: 1 in]
        n289 = invoke class="App" method="Clipboard.Write"("Param 0"=w465) -> ()  [unwired: 3 in, 4 out]
      }
      frame "Exit" {
        n290 = Unbundle By Name(w478) -> ("IDs"=w480:i32[])
        n291 = for {
          tunnel: w480 -> [w481] mode=indexing
          n292 = call "close device.vi"("id"=w481) -> ()  [unwired: 8 in, 3 out]
        }
        n293 = Open Application Reference(8:errorcluster {"status"=FALSE, "code"=0, "source"=""} ("error in (no error)")) -> (0:w471:errorcluster, 3:w472:refnum<vi>)  [unwired: 3 in]
        n294 = property class="App"(reference=w472, error in=w471) -> ("App.Kind"=w475:T2)  [unwired: 2 out]
        n295 = Equal?(x=w475, y=T2."Run Time System" ("Application:Kind")) -> (x = y?=w473:bool)
        n296 = Quit LabVIEW(quit? (T)=w473) -> ()
      }
    }
  }
